vi "Image Display Is ROI Selected.vi"(8 "Error In":errorcluster, 11 "Image Control Refnum":T2) -> (0 "Error Out":errorcluster, 1 "ROI":T1, 2 "Is ROI Selected?":bool)   [LabVIEW 2021, in "Image.lvlib"]
uses:
  Image.lvlib
  Image Control Refnum.ctl
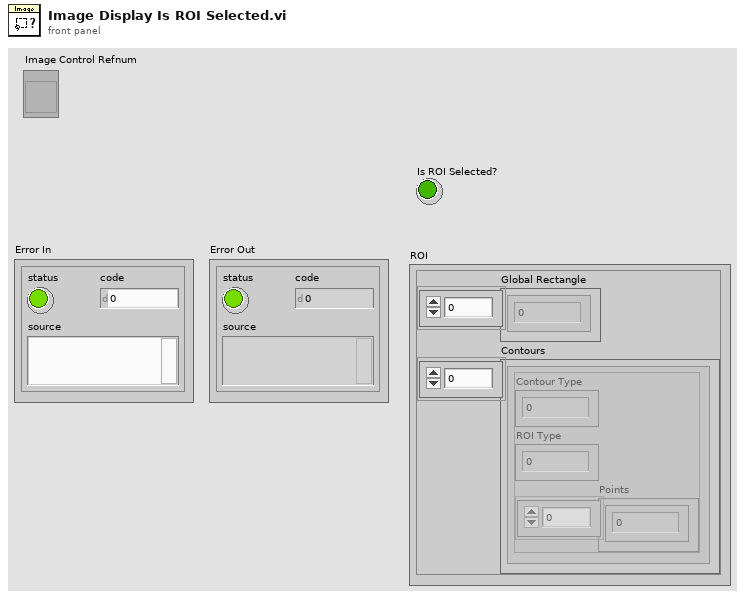
[diagram p1: front panel]
types:
  T1 = cluster{"Global Rectangle":i32[], "Contours":cluster{"Contour Type":u32, "ROI Type":u32, "Points":i32[]}[]}
  T2 = typedef "Image.lvlib/Image Control Refnum.ctl" = refnum<vi>
  T3 = cluster{"Contour Type":u32, "ROI Type":u32, "Points":i32[]}[]
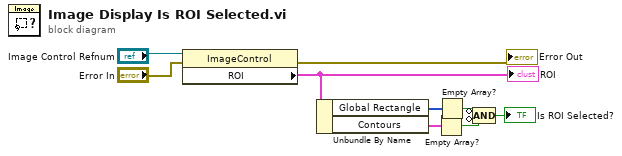
[diagram p0: block diagram]
diagram:
  n1 = property class="ImageControl"(reference="Image Control Refnum", error in="Error In") -> (error out=→"Error Out":errorcluster, "ROI"=w7:T1)  [unwired: 1 out]
  "ROI" <- w7
  n2 = Unbundle By Name(w7) -> ("Global Rectangle"=w6:i32[], "Contours"=w5:T3)
  n3 = Empty Array?(array=w5) -> (empty?=w3:bool)
  n4 = Empty Array?(array=w6) -> (empty?=w4:bool)
  n5 = Compound Arithmetic op=AND(invert w4, invert w3) -> (→"Is ROI Selected?":bool)
